vi "BroadcastSettings.vi"(8 "Error In":errorcluster, 11 "AutoData":T1) -> (0 "Error Out":errorcluster, 3 "AutoData out":T1)   [LabVIEW 2019, in "AutoMode.lvlib"]
uses:
  AutoMode.lvlib
  Cluster - AutoModeData.ctl
  MainController/Cluster - TestSettings.ctl
  MainController/Cluster - HardwareConfiguration.ctl
  MainController/Cluster - TestResults.ctl
  Cluster - AutoModeMessage.ctl
  Enum - AutoModeState.ctl
  MainController/Cluster - MainControllerMessage.ctl
  MainController/Enum - MainState.ctl
  MainController/MainController.lvlib
  Utilites/Utilities.lvlib
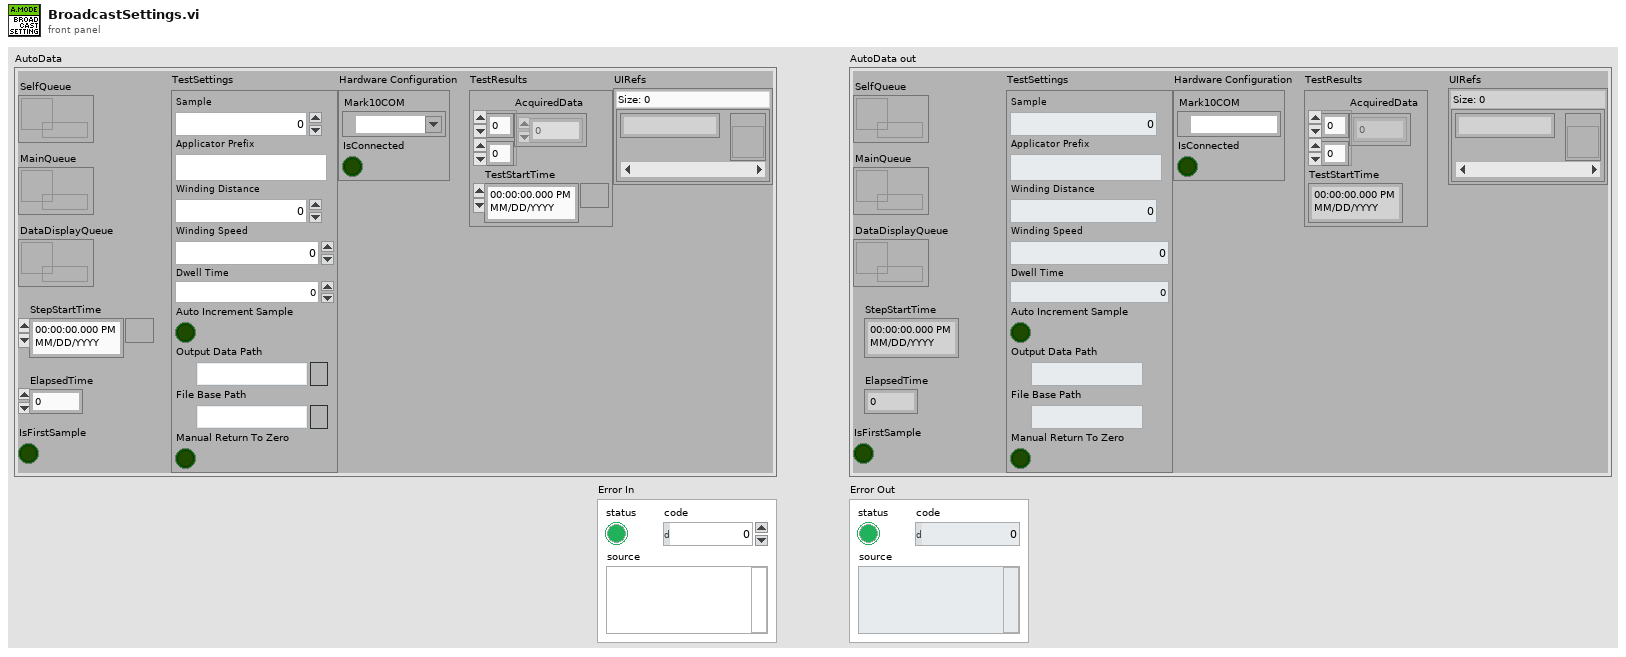
[diagram p1: front panel]
types:
  T1 = typedef "AutoMode.lvlib/Cluster - AutoModeData.ctl" = cluster{"DataDisplayQueue":refnum<queue>, "StepStartTime":timestamp, "TestSettings":T2, "Hardware Configuration":T3, "TestResults":T4, "ElapsedTime":dbl, "IsFirstSample":bool, "UIRefs":map{string, refnum<vi>}, "SelfQueue":refnum<queue>, "MainQueue":refnum<queue>}
  T2 = typedef "MainController.lvlib/Cluster - TestSettings.ctl" = cluster{"Sample":u32, "Applicator Prefix":string, "Winding Distance":dbl, "Winding Speed":dbl, "Dwell Time":dbl, "Auto Increment Sample":bool, "Output Data Path":path, "File Base Path":path, "Manual Return To Zero":bool}
  T3 = typedef "MainController.lvlib/Cluster - HardwareConfiguration.ctl" = cluster{"Mark10COM":refnum<visa-resource-name>, "IsConnected":bool}
  T4 = typedef "MainController.lvlib/Cluster - TestResults.ctl" = cluster{"AcquiredData":dbl[][], "TestStartTime":timestamp}
  T5 = typedef "MainController.lvlib/Enum - MainState.ctl" = enum16{"Initialize", "InitUIRefs", "LaunchSettings", "LaunchAutoMode", "LaunchManualMode", "LaunchTestReport", "ConnectHardware", "DisconnectHardware", "HiliteNavItems", "StartAutoMode", "PauseAutoMode", "StopAutoMode", "ShowFlyout", "HideFlyout", "BroadcastSettings", "PickupTestSettings", "BroadcastHW", "AutoTestDone", "DAQStatus", "UpdateCommandBar", "Error", "RecieveError", "Exit"}
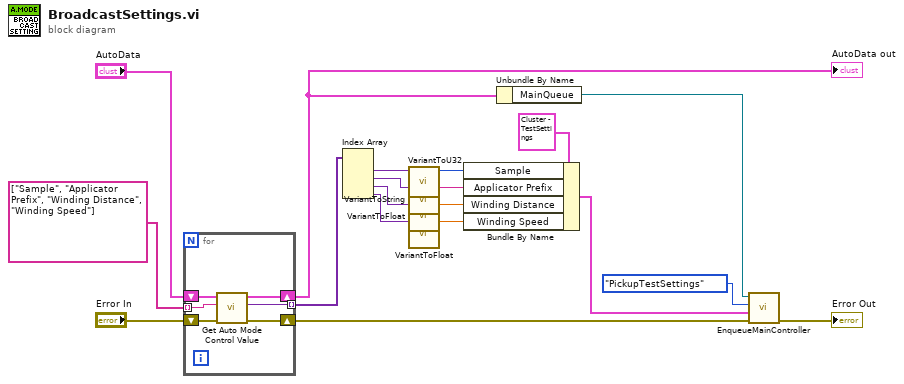
[diagram p0: block diagram]
diagram:
  n1 = for {
    shift-right: [w24] -> w13
    shift-left: "Error In" -> [w25]
    shift-right: [w22] -> w11
    shift-left: "AutoData" -> [w23]
    tunnel: string[] ["Sample", "Applicator Prefix", "Winding Distance", "Winding Speed"] ("key") -> [w21] mode=indexing
    tunnel: [w20] -> w9 mode=indexing
    n2 = call "Get Auto Mode Control Value.vi"("Error In"=w25, "key"=w21, "AutoData"=w23) -> ("Error Out"=w24:errorcluster, "Value"=w20:variant, "AutoData out"=w22:T1)  [unwired: 6 in]
  }
  "AutoData out" <- w11
  n3 = Index Array(array=w9) -> (element #1=w8:variant, element #2=w6:variant, element #3=w3:variant, element #4=w4:variant)  [unwired: 4 in]
  n4 = call "VariantToU32.vi"("Variant"=w8) -> ("Value"=w7:u32)  [unwired: 9 in, 1 out]
  n5 = call "VariantToString.vi"("Variant"=w6) -> ("Value"=w5:string)  [unwired: 9 in, 1 out]
  n6 = call "VariantToFloat.vi"("Variant"=w3) -> ("Value"=w1:dbl)  [unwired: 9 in, 1 out]
  n7 = call "VariantToFloat.vi"("Variant"=w4) -> ("Value"=w2:dbl)  [unwired: 9 in, 1 out]
  n8 = Bundle By Name(cluster=T2 {"Sample"=0, "Applicator Prefix"="", "Winding Distance"=0.0, "Winding Speed"=0.0, "Dwell Time"=0.0, "Auto Increment Sample"=FALSE, "Output Data Path"=path "", "File Base Path"=path "", "Manual Return To Zero"=FALSE} ("TestSettings"), "Sample"=w7, "Applicator Prefix"=w5, "Winding Distance"=w1, "Winding Speed"=w2) -> (w18:T2)
  n9 = Unbundle By Name(w11) -> ("MainQueue"=w16:refnum<queue>)
  n10 = call "EnqueueMainController.vi"("error in (no error)"=w13, "Data"=w18, "Message"=Enum_-_MainState."PickupTestSettings", "MainQueue"=w16) -> ("error out"=→"Error Out":errorcluster)  [unwired: 5 in, 2 out]
